vi "Medidor_File (2).vi"() -> (0 "Waveform Graph Voltage  2":dynamicdata(graph), 1 "Waveform Graph Current 1":dynamicdata(graph), 2 "Waveform Graph Voltage 1":dynamicdata(graph), 3 "Waveform Graph Current 2":dynamicdata(graph), 4 "Waveform Graph Voltage  3":dynamicdata(graph), 5 "Waveform Graph Current 3":dynamicdata(graph))   [LabVIEW 2020]
panel:
  out "Volatage and Current Phase 3":string[][](table)
  out "Current Phase 3 (A)":string[][](table)
  out "Voltage Phase 3 (V)":string[][](table)
  out "Volatage and Current Phase 2":string[][](table)
  out "Current Phase 2 (A)":string[][](table)
  out "Voltage Phase 2 (V)":string[][](table)
  out "Volatage and Current Phase 1":string[][](table)
  out "Current Phase 1 (A)":string[][](table)
  out "Voltage Phase 1 (V)":string[][](table)
  out "timestamp":string[][](table)
  out "Waveform Graph timestamp":dynamicdata(graph)
  out "Waveform Graph":dynamicdata(graph)
  out "All Data":string[][](table)
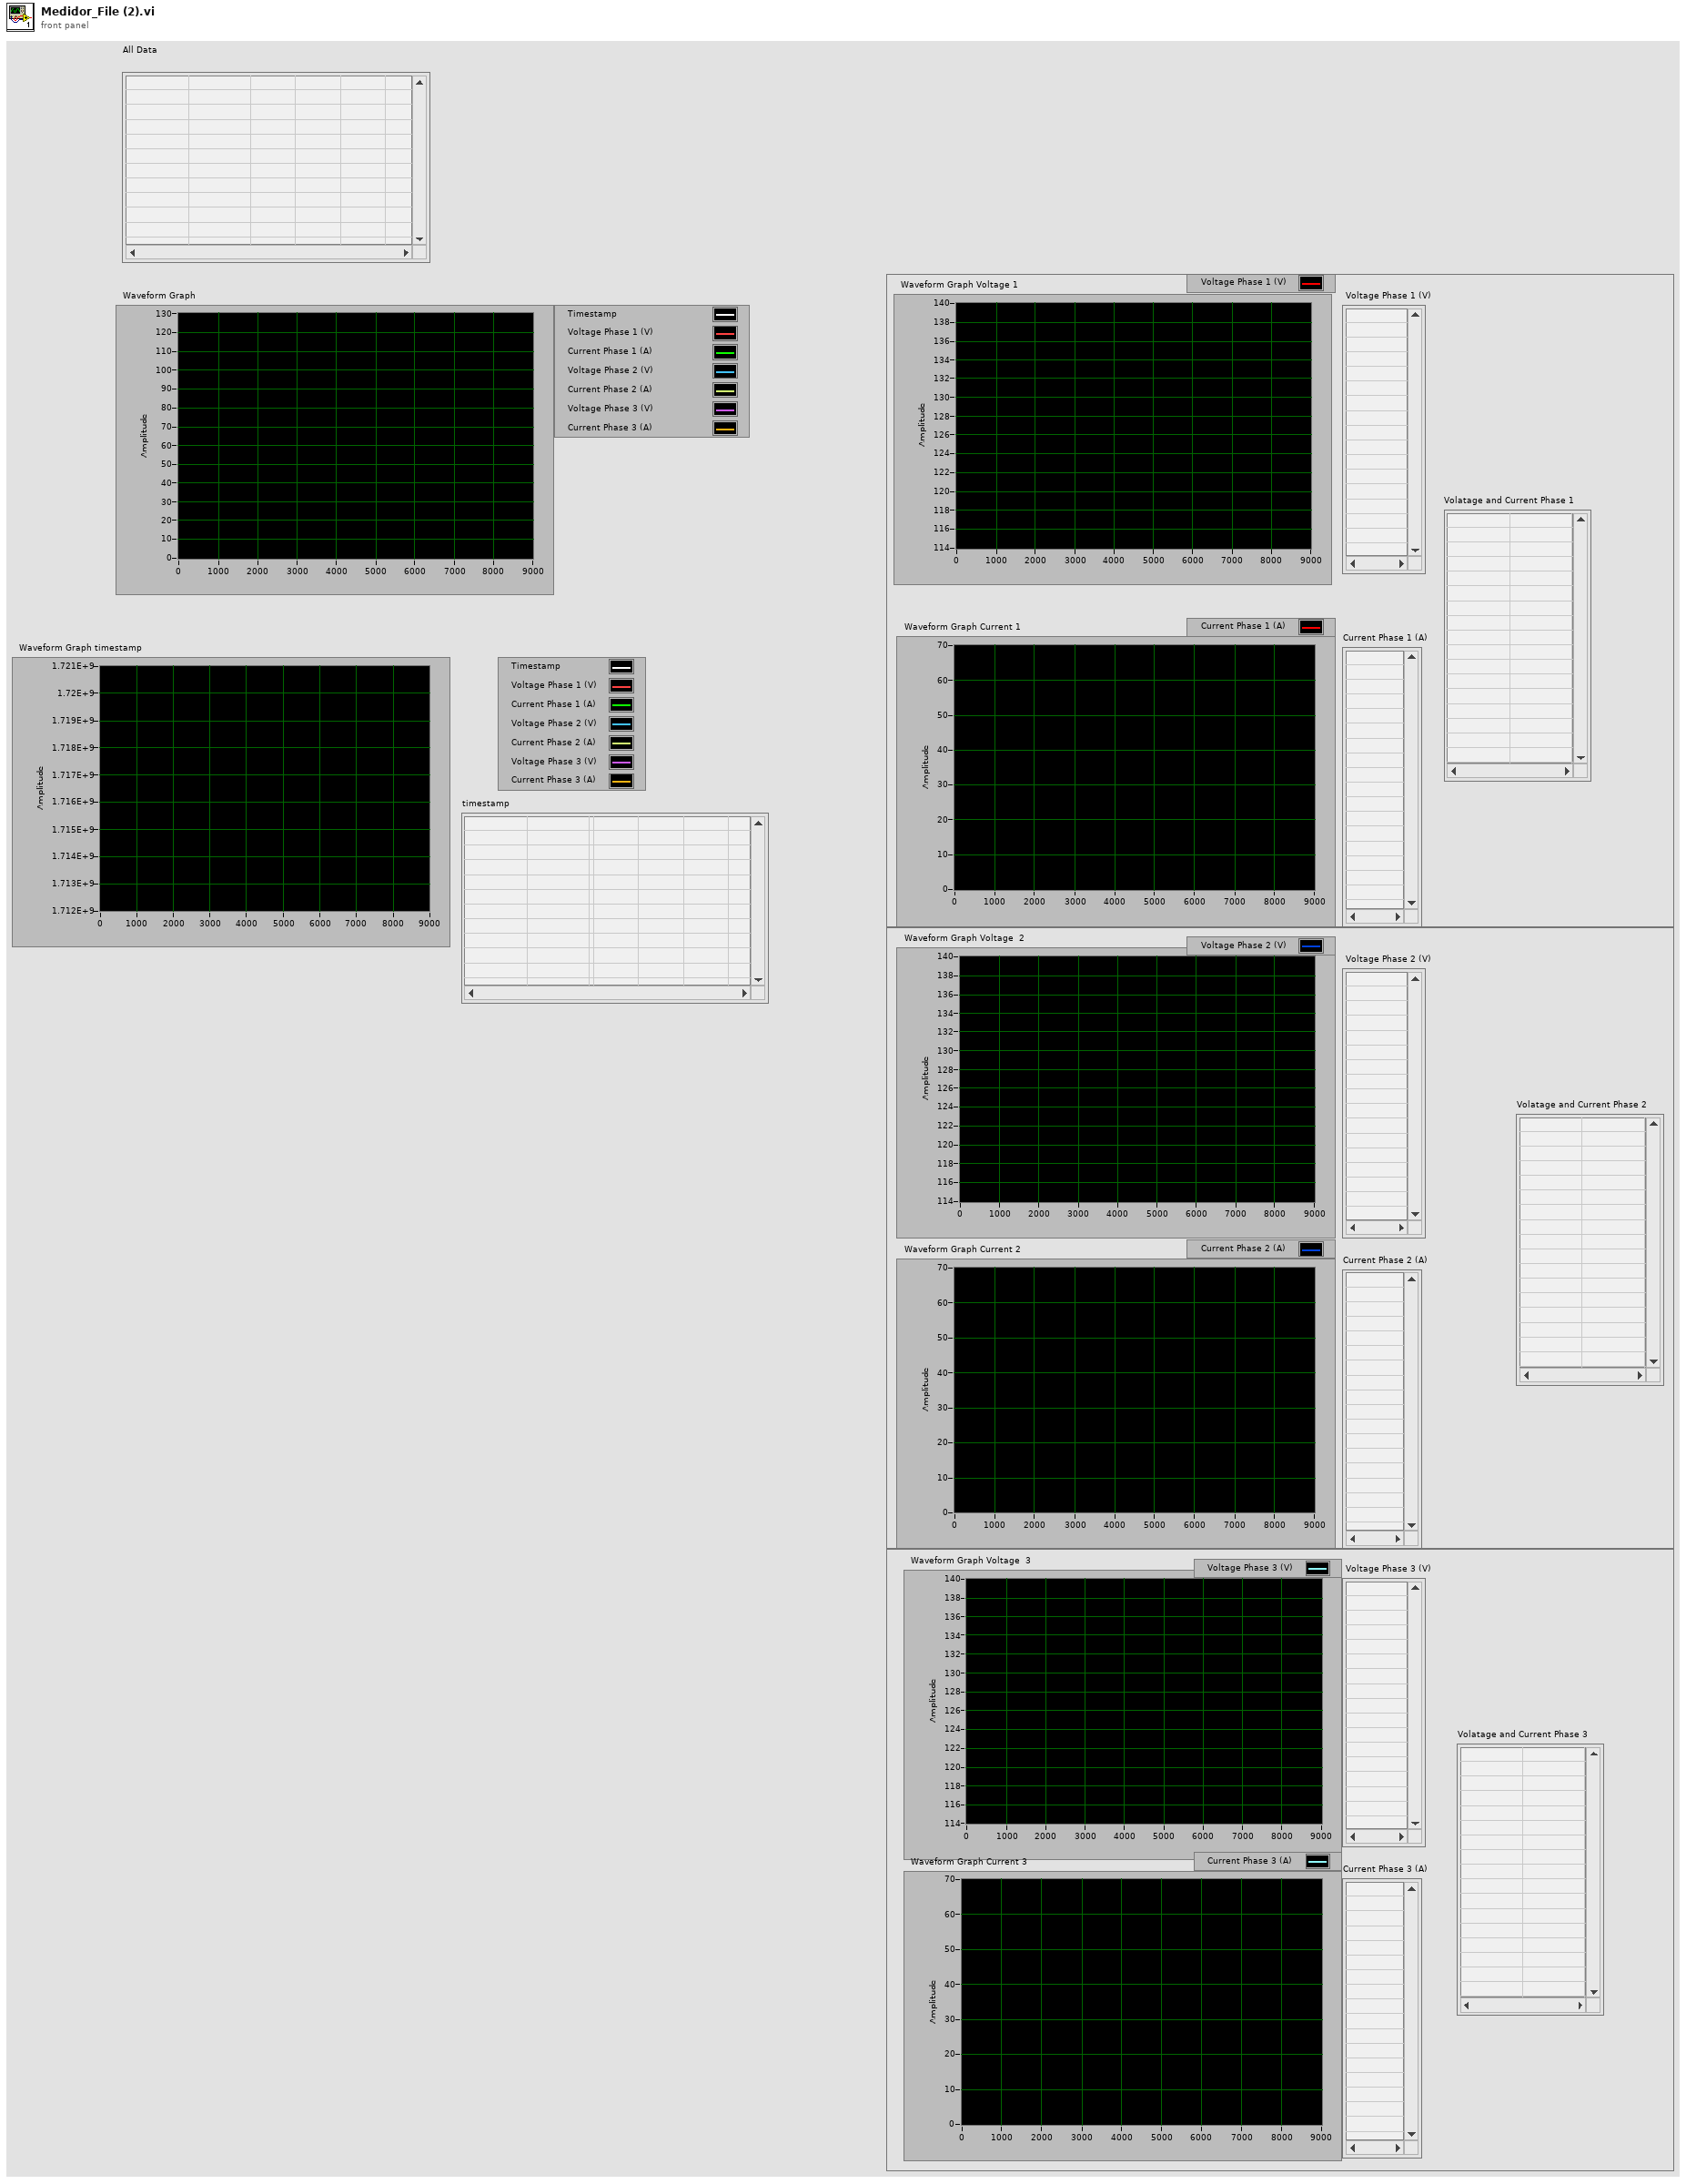
[diagram p1: front panel]
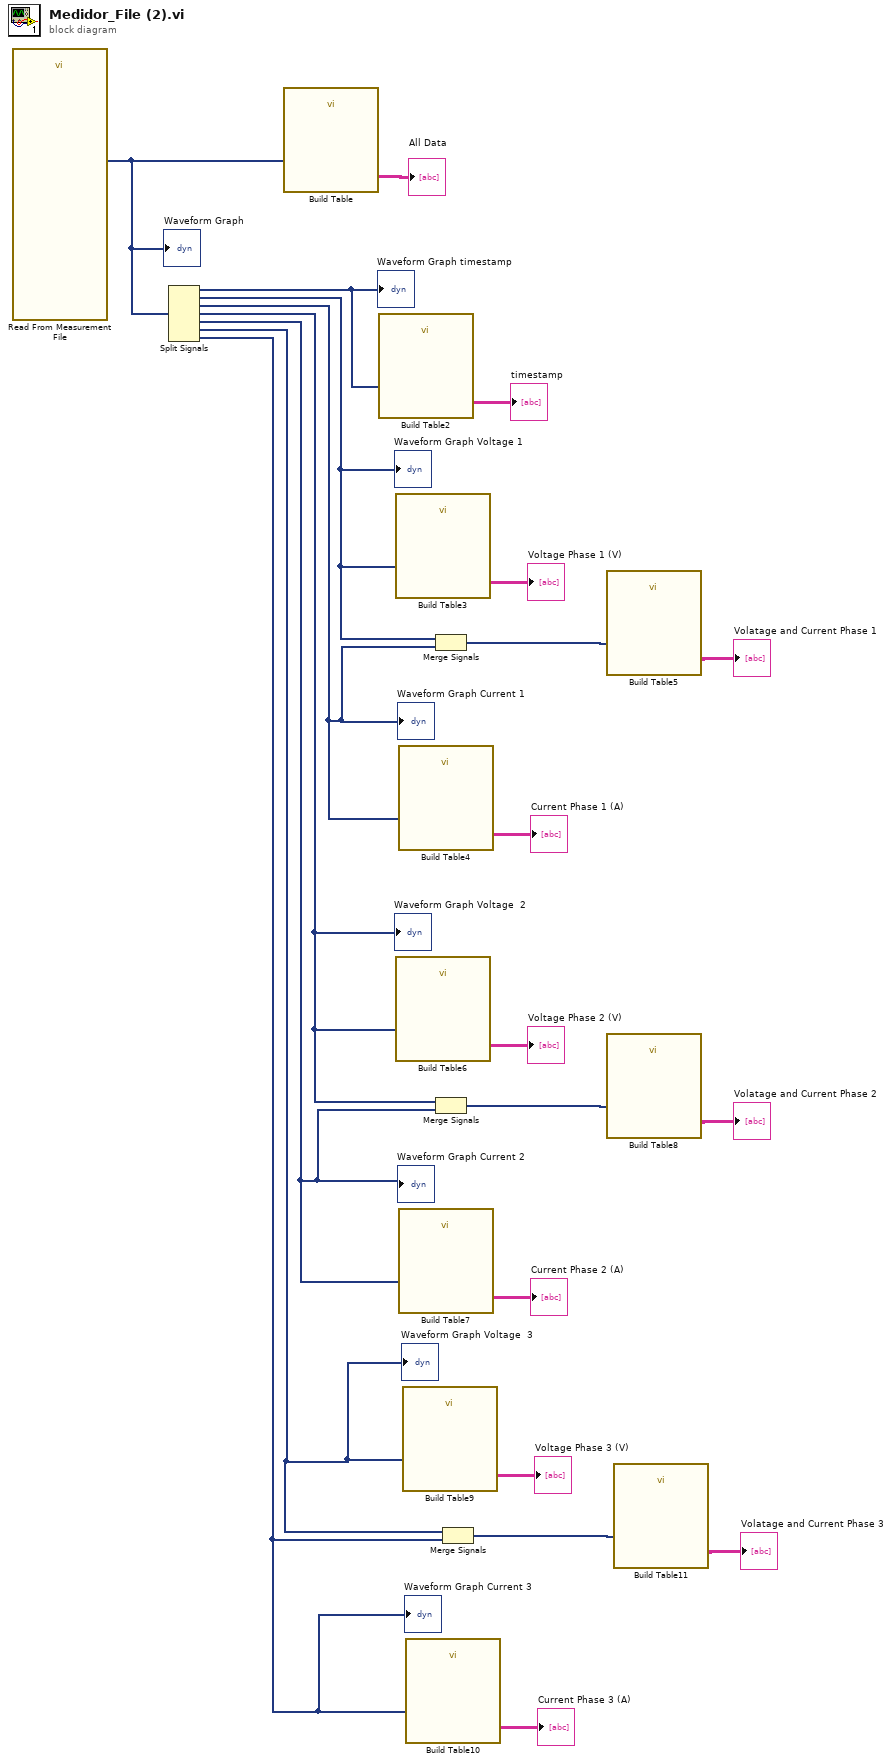
[diagram p0: block diagram]
diagram:
  n1 = call "Read From Measurement File"() -> ("Signals"=w21:dynamicdata)  [unwired: 6 in, 5 out]
  "Waveform Graph" <- w21
  n2 = Split Signals(w21) -> (w19:dynamicdata, w16:dynamicdata, w15:dynamicdata, w8:dynamicdata, w7:dynamicdata, w2:dynamicdata, w1:dynamicdata)  [unwired: 7 in]
  "Waveform Graph timestamp" <- w19
  "Waveform Graph Voltage 1" <- w16
  "Waveform Graph Current 1" <- w15
  "Waveform Graph Voltage  2" <- w8
  "Waveform Graph Current 2" <- w7
  "Waveform Graph Voltage  3" <- w2
  "Waveform Graph Current 3" <- w1
  n3 = call "Build Table"("Signals"=w21) -> ("Table"=→"All Data":string[][])  [unwired: 4 in, 6 out]
  n4 = call "Build Table2"("Signals"=w19) -> ("Table"=→"timestamp":string[][])  [unwired: 4 in, 6 out]
  n5 = call "Build Table3"("Signals"=w16) -> ("Table"=→"Voltage Phase 1 (V)":string[][])  [unwired: 4 in, 6 out]
  n6 = call "Build Table6"("Signals"=w8) -> ("Table"=→"Voltage Phase 2 (V)":string[][])  [unwired: 4 in, 6 out]
  n7 = call "Build Table4"("Signals"=w15) -> ("Table"=→"Current Phase 1 (A)":string[][])  [unwired: 4 in, 6 out]
  n8 = call "Build Table7"("Signals"=w7) -> ("Table"=→"Current Phase 2 (A)":string[][])  [unwired: 4 in, 6 out]
  n9 = call "Build Table9"("Signals"=w2) -> ("Table"=→"Voltage Phase 3 (V)":string[][])  [unwired: 4 in, 6 out]
  n10 = call "Build Table10"("Signals"=w1) -> ("Table"=→"Current Phase 3 (A)":string[][])  [unwired: 4 in, 6 out]
  n11 = Merge Signals(w16, w15) -> (w13:dynamicdata)
  n12 = Merge Signals(w8, w7) -> (w9:dynamicdata)
  n13 = Merge Signals(w2, w1) -> (w3:dynamicdata)
  n14 = call "Build Table5"("Signals"=w13) -> ("Table"=→"Volatage and Current Phase 1":string[][])  [unwired: 4 in, 6 out]
  n15 = call "Build Table8"("Signals"=w9) -> ("Table"=→"Volatage and Current Phase 2":string[][])  [unwired: 4 in, 6 out]
  n16 = call "Build Table11"("Signals"=w3) -> ("Table"=→"Volatage and Current Phase 3":string[][])  [unwired: 4 in, 6 out]
